vi "Write String Array (2D).vi"(8 "error in":errorcluster, 10 "Value":string[][](array[string]), 11 "String Array (2D) Ref in":refnum<vi>) -> (0 "error out":errorcluster, 3 "String Array (2D) Ref out":refnum<vi>)   [LabVIEW 2020, in "G-Unicode.lvlib"]
uses:
  G-Unicode.lvlib
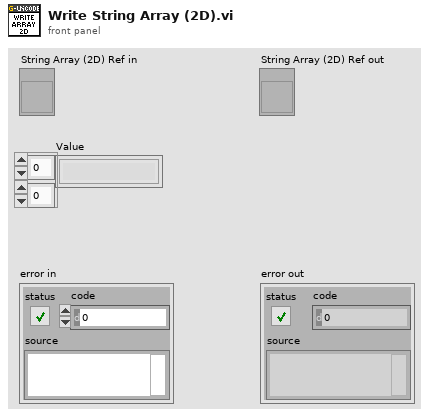
[diagram p1: front panel]
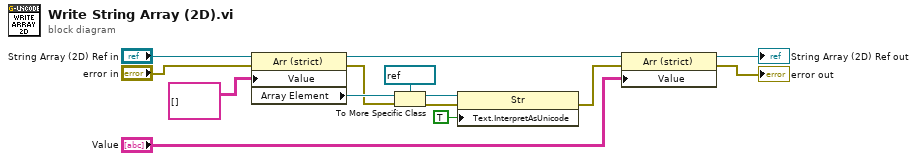
[diagram p0: block diagram]
diagram:
  n1 = property class="Arr (strict)"(reference="String Array (2D) Ref in", error in="error in", "Value"=string[][] []) -> (reference out=w6:refnum<vi>, error out=w12:errorcluster, "Array Element"=w13:refnum<vi>)
  n2 = To More Specific Class(target class=refnum<vi> refnum ("String"), reference=w13, error in=w12) -> (specific class reference=w11:refnum<vi>, error out=w9:errorcluster)
  n3 = property class="Str"(reference=w11, error in=w9, "Text.InterpretAsUnicode"=TRUE ("Text.Interpret As Unicode")) -> (error out=w4:errorcluster)  [unwired: 1 out]
  n4 = property class="Arr (strict)"(reference=w6, error in=w4, "Value"="Value") -> (reference out=→"String Array (2D) Ref out":refnum<vi>, error out=→"error out":errorcluster)
